vi "Read Payload.vi"(11 "ControlPacket in":refnum<class "ControlPacket.lvclass">) -> (2 "Payload":u8[](array[numeric]) format="%08b", 3 "ControlPacket out":refnum<class "ControlPacket.lvclass">)   [LabVIEW 2013, in "MQTT_Control_Packets.lvlib" / "ControlPacket.lvclass"]
uses:
  ControlPacket.lvclass
  ControlPacket.lvclass/ControlPacket.ctl
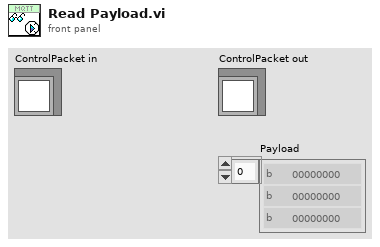
[diagram p1: front panel]
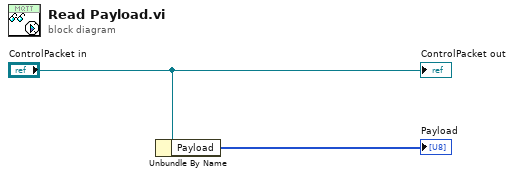
[diagram p0: block diagram]
diagram:
  n1 = Unbundle By Name("ControlPacket in") -> ("Payload"=→"Payload":u8[])
  "ControlPacket out" <- "ControlPacket in"
